vi "readFromXML.vi"(8 "error in (no error)":errorcluster, 10 "XML in":string="<DifftrackRADec>\n<dDec_ArcsPS>12.2</dDec_ArcsPS>\n<dRA_sps>112.2</dRA_sps>\n</DifftrackRADec>", 11 "DifftrackRADec in":refnum<class "DifftrackRADec.lvclass">) -> (0 "error out":errorcluster, 3 "DifftrackRADec out":refnum<class "DifftrackRADec.lvclass">)   [LabVIEW 2022 SP3, in "TCSDataDefinitions.lvlib" / "TCSCommand.lvlib" / "TargetConfiguration.lvlib" / "Target.lvlib" / "DifftrackRADec.lvclass"]
uses:
  DifftrackRADec.lvclass
  <userlib>/Common/UnitsAndXML/FlattenItemWithUnitToXML/FlattenAngularVelocityToXML/AngularVelocityUnit.ctl
  DifftrackRADec.lvclass/DifftrackRADec.ctl
  Difftrack.lvclass
  <userlib>/Common/UnitsAndXML/UnitsAndXML.lvlib
  <userlib>/Common/XML/XMLParser/XMLParser.lvclass
panel:
  out "dRA_sps":dbl=112.2
  out "dDec_ArcsPS":dbl[unit]=5.9147269095363384e-05
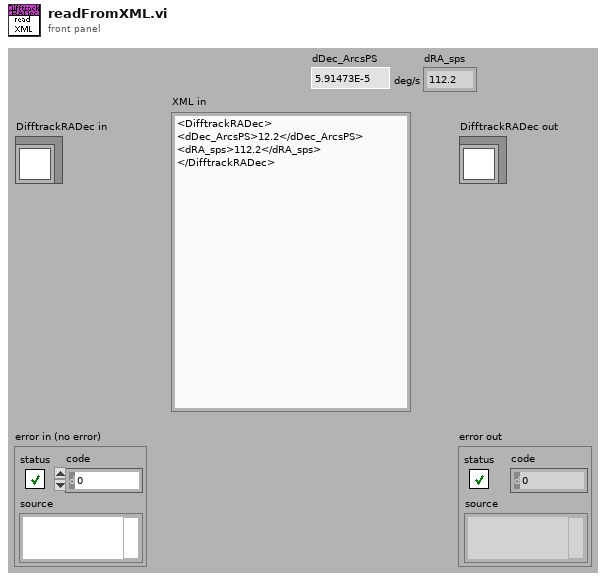
[diagram p1: front panel]
types:
  T1 = typedef "UnitsAndXML.lvlib/AngularVelocityUnit.ctl" = enum16{"\"/a", "deg/s", "\"/s"}
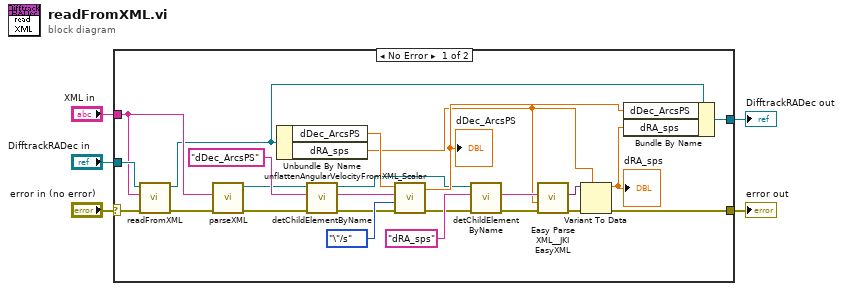
[diagram p0: block diagram]
diagram:
  n1 = case shown="No Error" "error in (no error)" {
    selector: "error in (no error)" -> [w24 w30]
    tunnel: [w9 w30] -> w5
    tunnel: [w19 w31] -> w4
    tunnel: "XML in" -> [w28 _]
    tunnel: "DifftrackRADec in" -> [w29 w31]
    frame No Error {
      n2 = call-parent "readFromXML.vi"("error in (no error)"=w24, "XML in"=w28, "Difftrack in"=w29) -> ("error out"=w23:errorcluster, "Difftrack out"=w20:refnum<class "DifftrackRADec.lvclass">)  [unwired: 7 in]
      n3 = call <userlib>:"parseXML.vi"("error in (no error)"=w23, "XMLString in"=w28) -> ("error out"=w27:errorcluster, "Element out"=w7:refnum<class "XMLParser.lvclass">)  [unwired: 8 in]
      n4 = Unbundle By Name(w20) -> ("dDec_ArcsPS"=w21:dbl[unit], "dRA_sps"=w11:dbl)
      n5 = call <userlib>:"detChildElementByName.vi"("error in (no error)"=w27, "childName"="dDec_ArcsPS" ("ChildName"), "Element in"=w7) -> ("error out"=w8:errorcluster, "childXML"=w22:string, "Element out"=w6:refnum<class "XMLParser.lvclass">)  [unwired: 5 in, 1 out]
      n6 = call <userlib>:"unflattenAngularVelocityFromXML_Scalar.vi"("error in (no error)"=w8, "angularVelocityUnitInXML"=AngularVelocityUnit."\"/s", "xmlString"=w22, "angularVelocityForType"=w21) -> ("error out"=w16:errorcluster, "angularVelocity"=w18:dbl[unit])  [unwired: 6 in]
      "dDec_ArcsPS" <- w18
      n7 = call <userlib>:"detChildElementByName.vi"("error in (no error)"=w16, "childName"="dRA_sps" ("ChildName"), "Element in"=w6) -> ("error out"=w15:errorcluster, "childXML"=w14:string)  [unwired: 5 in, 2 out]
      n8 = call <vilib>:"Easy Parse XML__JKI EasyXML.vi"("error in (no error)"=w15, "LabVIEW Data (Type)"=w11, "XML String"=w14) -> ("error out"=w13:errorcluster, "LabVIEW Data"=w12:variant)  [unwired: 7 in]
      n9 = Variant To Data(error in=w13, type=w11, Variant=w12) -> (data=w10:dbl, error out=w9:errorcluster)
      "dRA_sps" <- w10
      n10 = Bundle By Name(cluster=w20, "dDec_ArcsPS"=w18, "dRA_sps"=w10) -> (w19:refnum<class "DifftrackRADec.lvclass">)
    }
    frame Error {
    }
  }
  "error out" <- w5
  "DifftrackRADec out" <- w4
